vi "Write Data.vi"(7 "SPI Peripheral":refnum<class "SPI Peripheral.lvclass">, 8 "error in (no error)":errorcluster, 10 "Write Data":string, 11 "Session In":refnum<class "Session.lvclass">) -> (0 "error out":errorcluster, 3 "Session Out":refnum<class "Session.lvclass">)   [LabVIEW 2020, in "CTI.lvlib" / "SPI Peripheral.lvclass"]
uses:
  SPI Peripheral.lvclass
  Session/Session.lvclass
  SPI Peripheral.lvclass/SPI Peripheral.ctl
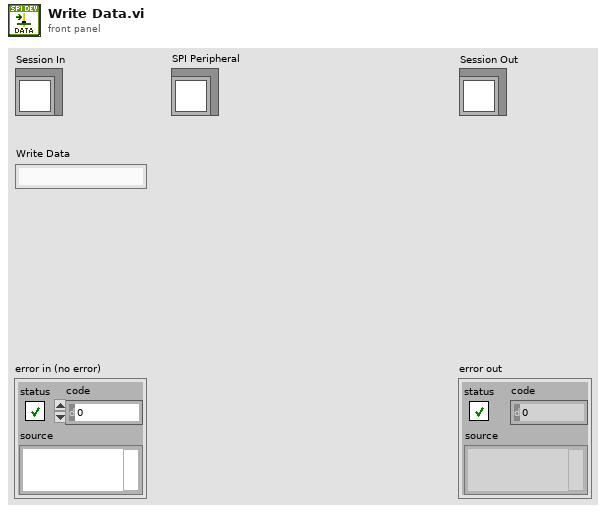
[diagram p1: front panel]
types:
  T1 = typedef "CTI.lvlib/SPI Number.ctl" = i8
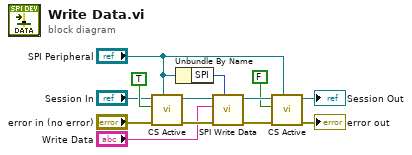
[diagram p0: block diagram]
diagram:
  n1 = call "CS Active.vi"("SPI Peripheral in"="SPI Peripheral", "error in (no error)"="error in (no error)", "CS Active"=TRUE, "Session In"="Session In") -> ("error out"=w11:errorcluster, "Session Out"=w9:refnum<class "Session.lvclass">)  [unwired: 6 in]
  n2 = Unbundle By Name("SPI Peripheral") -> ("SPI"=w10:T1)
  n3 = call "SPI Write Data.vi"("SPI #"=w10, "error in (no error)"=w11, "Data"="Write Data", "Session in"=w9) -> ("error out"=w12:errorcluster, "Session out"=w13:refnum<class "Session.lvclass">)  [unwired: 6 in]
  n4 = call "CS Active.vi"("SPI Peripheral in"="SPI Peripheral", "error in (no error)"=w12, "CS Active"=FALSE, "Session In"=w13) -> ("error out"=→"error out":errorcluster, "Session Out"=→"Session Out":refnum<class "Session.lvclass">)  [unwired: 6 in]
